vi "close all.vi"(8 "error in (no error)":errorcluster, 11 "p2p vst in":refnum<class "p2p vst.lvclass">) -> (0 "error out":errorcluster, 3 "p2p vst out":refnum<class "p2p vst.lvclass">)   [LabVIEW 2021, in "p2p vst.lvclass"]
uses:
  p2p vst.lvclass
  p2p vst.lvclass/p2p vst.ctl
  <vilib>/FPGAPlugInAG/Dynamic/niLvFpga_Close_Dynamic.vi
  <vilib>/rvi/interface/nirviCloseFPGA/nirviCloseFPGA.xnode
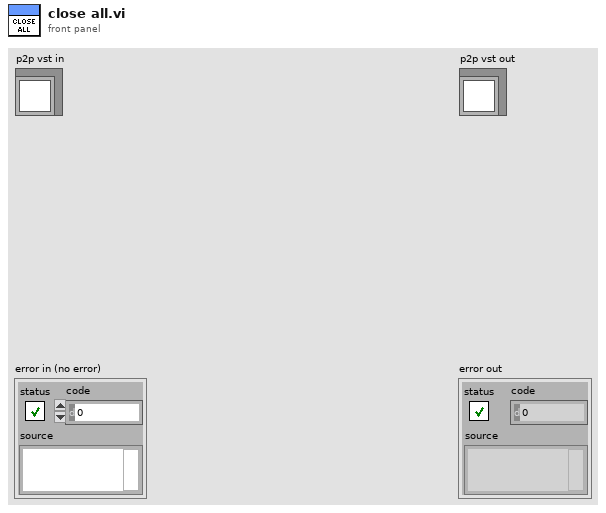
[diagram p1: front panel]
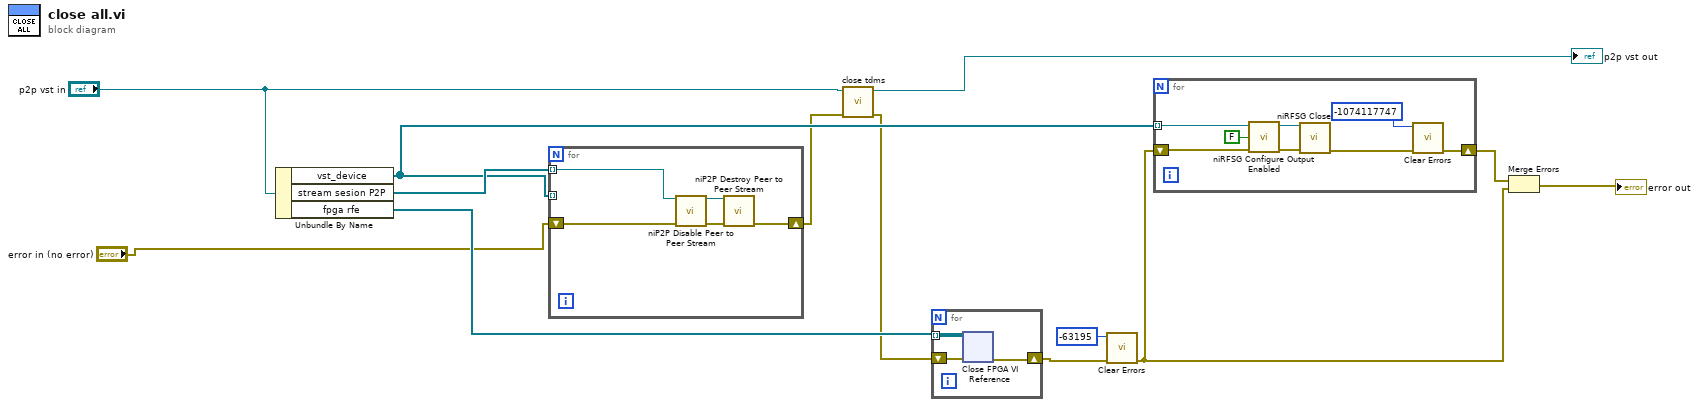
[diagram p0: block diagram]
diagram:
  n1 = Unbundle By Name("p2p vst in") -> ("vst_device"=w9:refnum<k15>[], "stream sesion P2P"=w10:refnum<k20>[], "fpga rfe"=w13:refnum<k20>[])
  n2 = for {
    tunnel: w10 -> [w15] mode=indexing
    shift-right: [w16] -> w2
    shift-left: "error in (no error)" -> [w14]
    tunnel: w9 -> [_] mode=indexing
    n3 = call <vilib>:"niP2P Disable Peer to Peer Stream.vi"("stream session"=w15, "error in (no error)"=w14) -> ("stream session out"=w18:refnum<k20>, "error out"=w17:errorcluster)  [unwired: 12 in]
    n4 = call <vilib>:"niP2P Destroy Peer to Peer Stream.vi"("stream session"=w18, "error in (no error)"=w17) -> ("error out"=w16:errorcluster)  [unwired: 13 in]
  }
  n5 = call-dynamic "close tdms.vi"("error in (no error)"=w2, "device_type in"="p2p vst in") -> ("error out"=w1:errorcluster, "device_type out"=→"p2p vst out":refnum<class "p2p vst.lvclass">)  [unwired: 8 in]
  n6 = for {
    shift-right: [w20] -> w11
    shift-left: w1 -> [w21]
    tunnel: w13 -> [w19] mode=indexing
    n7 = xnode "Close FPGA VI Reference"("FPGA VI Reference In"=w19, "error in"=w21) -> ("error out"=w20:errorcluster)
  }
  n8 = call <vilib>:"Clear Errors.vi"("error in (no error)"=w11, "specific error code to clear (0: all)"=-63195) -> ("error out"=w8:errorcluster)  [unwired: 4 in, 1 out]
  n9 = for {
    tunnel: w9 -> [w29] mode=indexing
    shift-right: [w22] -> w7
    shift-left: w8 -> [w28]
    n10 = call <instrlib>:"niRFSG Configure Output Enabled.vi"("instrument handle"=w29, "output enabled"=FALSE, "error in"=w28) -> ("instrument handle out"=w26:refnum<k15>, "error out"=w27:errorcluster)  [unwired: 11 in]
    n11 = call <instrlib>:"niRFSG Close.vi"("instrument handle"=w26, "error in"=w27) -> ("error out"=w23:errorcluster)  [unwired: 13 in]
    n12 = call <vilib>:"Clear Errors.vi"("error in (no error)"=w23, "specific error code to clear (0: all)"=-1074117747) -> ("error out"=w22:errorcluster)  [unwired: 4 in, 1 out]
  }
  n13 = Merge Errors(w7, w8) -> (→"error out":errorcluster)
